vi "Alicat Simplified Driver Example_Setpoint.vi"() -> ()   [LabVIEW 2016]
doc: "Simplified example program for initializing the COM port, determining the data frame of an Alicat, acquiring the data of the same Alicat, and writing a setpoint to the same device. \n\nThis is a slightly more feature rich version of the Alicat Simplified Driver Example, and contains an example of a method for easily implementing fast setpoint writes."
panel:
  out "Measurement Data":T1
  in  "Setpoint":dbl format="%_4g"
  in  "Min. time between \nreadings [ms]":u32
  out "Elapsed Time [ms]":dbl caption="Elapsed Time (s)"
  in  "End Program":bool
  out "Error Text":string
  out "Error Present":bool
  out "Range Exceeded":bool
  in  "COM Port Settings":T2={"Unit ID"="A", "Baud Rate"=enum."19200", "VISA Sesssion In"="COM1"}
  # "Serial/Local setpoint should not be saved if setpoint changes more frequently than once per second (to avoid burning out the EEPROM memory with excessive writes). \n\nAdjust this setting using the \"Write Power-up Settings\" sub-VI."
  # "Totalizer Timer"
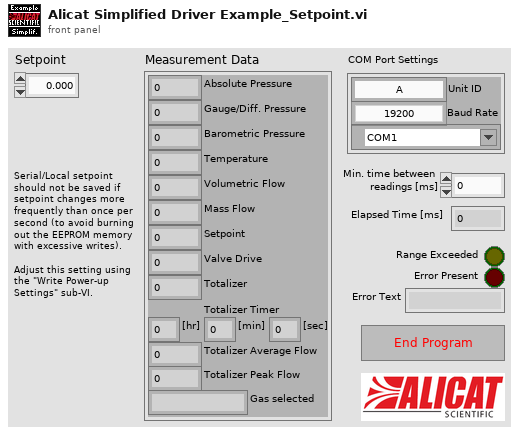
[diagram p1: front panel]
types:
  T1 = cluster{"Absolute Pressure":dbl, "Gauge/Diff. Pressure":dbl, "Barometric Pressure":dbl, "Temperature":dbl, "Volumetric Flow":dbl, "Mass Flow":dbl, "Setpoint":dbl, "Valve Drive":dbl, "Totalizer":dbl, "[hr]":dbl, "[min]":dbl, "[sec]":dbl, "Totalizer Average Flow":dbl, "Totalizer Peak Flow":dbl, "Gas selected":string}
  T2 = cluster{"Unit ID":string, "Baud Rate":enum8{"2400", "9600", "19200", "38400", "57600", "115200", "Unknown"}, "VISA Sesssion In":refnum<visa-resource-name>}
  T3 = cluster{"Absolute Pressure":bool, "Gauge/Diff. Pressure":bool, "Barometric Pressure":bool, "Temperature":bool, "Volumetric":bool, "Mass":bool, "Setpoint":bool, "Valve Drive":bool, "Totalizer":bool, "Totalizer Timer":bool, "Totalizer Average Flow":bool, "Totalizer Peak Flow":bool, "Gas Selected":bool, "Tot. Timer Format":u16}
  T4 = cluster{"Controller Full Scale":dbl, "Controller Select":u16, "Control Range":enum16{"Normal", "Inverted", "Bidirectional", "Unknown"}}
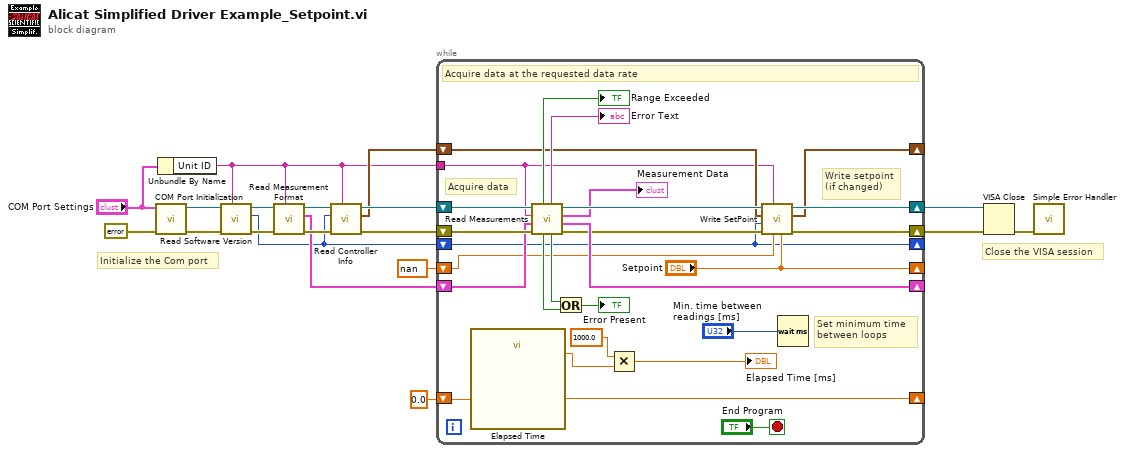
[diagram p0: block diagram]
diagram:
  # "Close the VISA session"
  # "Initialize the Com port"
  n1 = call "COM Port Initialization.vi"("error in (no error)"=errorcluster {"status"=FALSE, "code"=0, "source"=""}, "Communication Settings"="COM Port Settings") -> ("error out"=w5:errorcluster, "VISA Session Out"=w6:refnum<visa-resource-name>)  [unwired: 8 in]
  n2 = Unbundle By Name("COM Port Settings") -> ("Unit ID"=w4:string)
  n3 = call "Read Software Version.vi"("Unit ID (A)"=w4, "error in"=w5, "VISA Session In"=w6) -> ("error out"=w3:errorcluster, "Software Version"=w1:u8, "VISA Session Out"=w2:refnum<visa-resource-name>)  [unwired: 6 in]
  n4 = call "Read Measurement Format.vi"("Unit ID (A)"=w4, "error in"=w3, "VISA Session In"=w2) -> ("error out"=w13:errorcluster, "Data Frame Format"=w11:T3, "VISA Session Out"=w12:refnum<visa-resource-name>)  [unwired: 6 in]
  n5 = call "Read Controller Info.vi"("Unit ID (A)"=w4, "error in"=w13, "Software Version"=w1, "VISA Session In"=w12) -> ("error out"=w9:errorcluster, "Controller Info out"=w8:T4, "VISA Session Out"=w10:refnum<visa-resource-name>)  [unwired: 4 in, 1 out]
  n6 = while {
    shift-right: [w43] -> _
    shift-left: 0.0 ("Set Start Time (s)") -> [w46]
    shift-right: [w23] -> w14
    shift-left: w9 -> [w45]
    shift-right: [w30] -> w15
    shift-left: w10 -> [w44]
    tunnel: w4 -> [w25]
    shift-right: [w27] -> _
    shift-left: w11 -> [w42]
    shift-right: [w28] -> _
    shift-left: w8 -> [w29]
    shift-right: ["Setpoint"] -> _
    shift-left: nan ("Setpoint") -> [w26]
    shift-right: [w20] -> _
    shift-left: w1 -> [w20]
    stop <- "End Program" stop-if-true
    # "Write setpoint\n(if changed)"
    # "Set minimum time\nbetween loops"
    # "Acquire data"
    # "Acquire data at the requested data rate"
    n7 = call "Elapsed Time"("Set Start Time (s)"=w46) -> ("Get Start Time (s)"=w43:dbl, "Elapsed Time (s)"=w33:dbl)  [unwired: 11 in, 6 out]
    n8 = call "Read Measurements.vi"("error in"=w45, "Data Frame Format In"=w42, "Unit ID (A)"=w25, "VISA Session In"=w44) -> ("error out"=w24:errorcluster, "Data Frame Format Out"=w27:T3, "Data Cluster"=→"Measurement Data":T1, "VISA Session Out"=w31:refnum<visa-resource-name>, "Unknown Dataframe Info"=w41:bool, "Error/Overrange/Unknown String"=→"Error Text":string, "Error Present"=w40:bool, "Range Exceeded"=→"Range Exceeded":bool)
    n9 = Or(x=w41, y=w40) -> (x .or. y?=→"Error Present":bool)
    n10 = Multiply(x=1000.0 ("y"), y=w33) -> (x*y=→"Elapsed Time [ms]":dbl)
    n11 = call "Write SetPoint.vi"("Setpoint"="Setpoint", "Previous Setpoint"=w26, "Unit ID (A)"=w25, "error in"=w24, "Software Version"=w20, "Controller Info out"=w29, "VISA Session In"=w31) -> ("error out"=w23:errorcluster, "Controller Info out"=w28:T4, "VISA Session Out"=w30:refnum<visa-resource-name>)  [unwired: 1 in, 1 out]
    n12 = Wait (ms)(milliseconds to wait="Min. time between \nreadings [ms]") -> ()  [unwired: 1 out]
  }
  n13 = VISA Close(VISA resource name=w15, error in (no error)=w14) -> (error out=w16:errorcluster)
  n14 = call <vilib>:"Simple Error Handler.vi"("error in (no error)"=w16) -> ()  [unwired: 4 in, 5 out]
